vi "PH_SSAC.correct Frames.vi"(0 "i ref in":refnum<vi>, 5 "error in":errorcluster) -> (14 "i ref out":refnum<vi>, 19 "error out":errorcluster)   [LabVIEW 2014, in "PH_SSAC.lvlib"]
doc: "This VI checks the image size and corrects - if necessary - the size of the frames used for the main and the background signal."
uses:
  PH_SSAC.lvlib
  PH_SSAC.Signal Selector.ctl
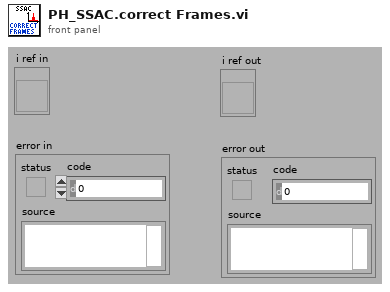
[diagram p1: front panel]
types:
  T1 = typedef "PH_SSAC.lvlib/PH_SSAC.Signal Selector.ctl" = enum16{"Main", "Background"}
  T2 = typedef "PH_SSAC.lvlib/PH_SSAC.i attribute.ctl" = cluster{"GUI Refs":cluster{"Delete":refnum<vi>, "Global On":refnum<vi>, "Cam Source":refnum<vi>, "Frame Main Signal":refnum<vi>, "Frame Background":refnum<vi>, "dt (Gauss smooth)":refnum<vi>, "Calibration Factor":refnum<vi>, "Background acquire":refnum<vi>, "Threshold":refnum<vi>, "Time evolution of mean pulse duration":refnum<vi>, "Mean Pulse Duration":refnum<vi>, "Main signal":refnum<vi>, "Current Pulse Duration":refnum<vi>, "Processed":refnum<vi>, "Saturation":refnum<vi>, "# for Average":refnum<vi>, "Position":refnum<vi>, "BG Status":refnum<vi>, "Save BG data":refnum<vi>, "Read BG Data":refnum<vi>, "Background Calibration Data":refnum<vi>}, "Images":cluster{"OP Image":T3, "GUI Image":T3, "PSDB Image":T3}, "Global On?":bool, "Frame Main":cluster{"x":u32, "dx":u32, "y":u32, "dy":u32}, "Frame Background":cluster{"x":u32, "dx":u32, "y":u32, "dy":u32}, "dt [fs]":dbl, "Calibration Factor [fs/pixel]":dbl, "Threshold":dbl, "Time evolution of mean pulse duration [fs]":dbl[], "Main Signal":cluster{"Time for Main":dbl[], "Signal":dbl[]}, "Processed":bool, "Current Pulse Duration [fs]":dbl, "# for Average":i32, "Position":i32, "Pulse Durations [fs]":dbl[], "BG":cluster{"Acquire?":bool, "Background Calibration Data":T4, "Save Data":bool}}
  T3 = typedef "IMAQ Image.ctl" = refnum<image>
  T4 = typedef "PH_SSAC.lvlib/PH_SSAC.Background Data.ctl" = cluster{"Date":string, "Time":string, "Frame Main":cluster{"x":u32, "dx":u32, "y":u32, "dy":u32}, "dt [fs]":dbl, "Calibration Factor [fs/pixel]":dbl, "Signal":dbl[], "Frame Background":cluster{"x":u32, "dx":u32, "y":u32, "dy":u32}}
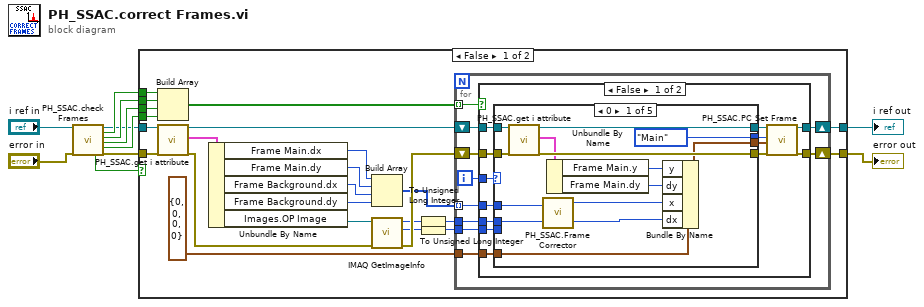
[diagram p0: block diagram]
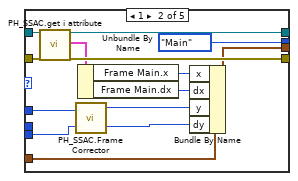
[diagram p2: hidden frame]
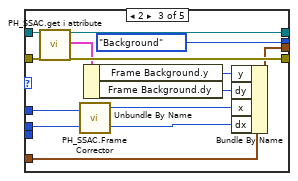
[diagram p3: hidden frame]
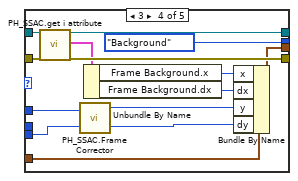
[diagram p4: hidden frame]
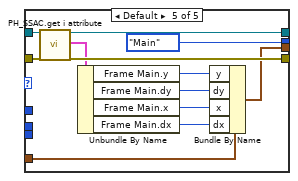
[diagram p5: hidden frame]
diagram:
  n1 = call "PH_SSAC.check Frames.vi"("i ref in"="i ref in", "error in"="error in") -> ("All ok?"=w1:bool, "i ref out"=w2:refnum<vi>, "x Dimension Main ok?"=w9:bool, "y Dimension Main ok?"=w8:bool, "x Dimension Background ok?"=w7:bool, "y Dimension Background ok?"=w6:bool, "error out"=w3:errorcluster)  [unwired: 11 in]
  n2 = case shown="False" w1 {
    tunnel: [w32 w130] -> w11
    tunnel: [w30 w129] -> w10
    tunnel: w9 -> [w20 _]
    tunnel: w8 -> [w19 _]
    tunnel: w7 -> [w18 _]
    tunnel: w6 -> [w17 _]
    tunnel: w3 -> [w16 w129]
    tunnel: w2 -> [w15 w130]
    frame False {
      n3 = Build Array(w20, w19, w18, w17) -> (w33:bool[])
      n4 = call "PH_SSAC.get i attribute.vi"("i ref in"=w15, "error in (no error)"=w16) -> ("i ref out"=w14:refnum<vi>, "i attribute"=w35:T2, "error out"=w13:errorcluster)  [unwired: 15 in]
      n5 = Unbundle By Name(w35) -> ("Frame Main.dx"=w29:u32, "Frame Main.dy"=w23:u32, "Frame Background.dx"=w22:u32, "Frame Background.dy"=w21:u32, "Images.OP Image"=w34:T3)
      n6 = Build Array(w29, w23, w22, w21) -> (w24:u32[])
      n7 = call "IMAQ GetImageInfo"("error in (no error)"=w13, "Image"=w34) -> ("error out"=w31:errorcluster, "Y Resolution"=w27:i32, "X Resolution"=w28:i32)  [unwired: 2 in, 5 out]
      n8 = To Unsigned Long Integer(number=w28) -> (unsigned 32bit integer=w26:u32)
      n9 = To Unsigned Long Integer(number=w27) -> (unsigned 32bit integer=w25:u32)
      n10 = for {
        tunnel: w33 -> [w41] mode=indexing
        shift-right: [w44] -> w32
        shift-left: w14 -> [w45]
        shift-right: [w42] -> w30
        shift-left: w31 -> [w43]
        tunnel: w26 -> [w39]
        tunnel: w24 -> [w38] mode=indexing
        tunnel: w25 -> [w37]
        tunnel: cluster{"x":u32, "dx":u32, "y":u32, "dy":u32} {"x"=0, "dx"=0, "y"=0, "dy"=0} ("Frame") -> [w36]
        i -> [w40]
        n11 = case shown="False" w41 {
          tunnel: w45 -> [w53 w128]
          tunnel: [w58 w128] -> w44
          tunnel: w43 -> [w55 w127]
          tunnel: [w57 w127] -> w42
          tunnel: w40 -> [w51 _]
          tunnel: w39 -> [w49 _]
          tunnel: w38 -> [w48 _]
          tunnel: w37 -> [w47 _]
          tunnel: w36 -> [w46 _]
          frame False {
            n12 = case shown="0" w51 {
              tunnel: [PH_SSAC.Signal_Selector."Main" ("Signal") PH_SSAC.Signal_Selector."Main" ("Signal") PH_SSAC.Signal_Selector."Background" ("Signal") PH_SSAC.Signal_Selector."Background" ("Signal") PH_SSAC.Signal_Selector."Main" ("Signal")] -> w56
              tunnel: w55 -> [w71 w85 w99 w113 w125]
              tunnel: [w70 w84 w98 w112 w124] -> w54
              tunnel: w53 -> [w69 w83 w97 w111 w123]
              tunnel: [w68 w82 w96 w110 w122] -> w52
              tunnel: [w67 w81 w95 w109 w121] -> w50
              tunnel: w49 -> [w62 _ w91 _ _]
              tunnel: w48 -> [w61 w77 w90 w105 _]
              tunnel: w47 -> [_ w76 _ w104 _]
              tunnel: w46 -> [w59 w73 w87 w101 w115]
              frame 0 {
                n13 = call "PH_SSAC.get i attribute.vi"("i ref in"=w69, "error in (no error)"=w71) -> ("i ref out"=w68:refnum<vi>, "i attribute"=w66:T2, "error out"=w70:errorcluster)  [unwired: 15 in]
                n14 = call "PH_SSAC.Frame Corrector.vi"("Image Dimension"=w62, "Frame Dimension"=w61) -> ("Corrected Frame Dimension"=w60:u32, "Corrected Frame Start Point"=w63:u32)
                n15 = Unbundle By Name(w66) -> ("Frame Main.y"=w65:u32, "Frame Main.dy"=w64:u32)
                n16 = Bundle By Name(cluster=w59, "y"=w65, "dy"=w64, "x"=w63, "dx"=w60) -> (w67:cluster{"x":u32, "dx":u32, "y":u32, "dy":u32})
              }
              frame 1 {
                n17 = call "PH_SSAC.get i attribute.vi"("i ref in"=w83, "error in (no error)"=w85) -> ("i ref out"=w82:refnum<vi>, "i attribute"=w80:T2, "error out"=w84:errorcluster)  [unwired: 15 in]
                n18 = call "PH_SSAC.Frame Corrector.vi"("Image Dimension"=w76, "Frame Dimension"=w77) -> ("Corrected Frame Dimension"=w74:u32, "Corrected Frame Start Point"=w75:u32)
                n19 = Unbundle By Name(w80) -> ("Frame Main.x"=w79:u32, "Frame Main.dx"=w78:u32)
                n20 = Bundle By Name(cluster=w73, "x"=w79, "dx"=w78, "y"=w75, "dy"=w74) -> (w81:cluster{"x":u32, "dx":u32, "y":u32, "dy":u32})
              }
              frame 2 {
                n21 = call "PH_SSAC.get i attribute.vi"("i ref in"=w97, "error in (no error)"=w99) -> ("i ref out"=w96:refnum<vi>, "i attribute"=w94:T2, "error out"=w98:errorcluster)  [unwired: 15 in]
                n22 = call "PH_SSAC.Frame Corrector.vi"("Image Dimension"=w91, "Frame Dimension"=w90) -> ("Corrected Frame Dimension"=w88:u32, "Corrected Frame Start Point"=w89:u32)
                n23 = Unbundle By Name(w94) -> ("Frame Background.y"=w93:u32, "Frame Background.dy"=w92:u32)
                n24 = Bundle By Name(cluster=w87, "y"=w93, "dy"=w92, "x"=w89, "dx"=w88) -> (w95:cluster{"x":u32, "dx":u32, "y":u32, "dy":u32})
              }
              frame 3 {
                n25 = call "PH_SSAC.get i attribute.vi"("i ref in"=w111, "error in (no error)"=w113) -> ("i ref out"=w110:refnum<vi>, "i attribute"=w108:T2, "error out"=w112:errorcluster)  [unwired: 15 in]
                n26 = call "PH_SSAC.Frame Corrector.vi"("Image Dimension"=w104, "Frame Dimension"=w105) -> ("Corrected Frame Dimension"=w102:u32, "Corrected Frame Start Point"=w103:u32)
                n27 = Unbundle By Name(w108) -> ("Frame Background.x"=w107:u32, "Frame Background.dx"=w106:u32)
                n28 = Bundle By Name(cluster=w101, "x"=w107, "dx"=w106, "y"=w103, "dy"=w102) -> (w109:cluster{"x":u32, "dx":u32, "y":u32, "dy":u32})
              }
              frame Default {
                n29 = call "PH_SSAC.get i attribute.vi"("i ref in"=w123, "error in (no error)"=w125) -> ("i ref out"=w122:refnum<vi>, "i attribute"=w120:T2, "error out"=w124:errorcluster)  [unwired: 15 in]
                n30 = Unbundle By Name(w120) -> ("Frame Main.y"=w119:u32, "Frame Main.dy"=w118:u32, "Frame Main.x"=w117:u32, "Frame Main.dx"=w116:u32)
                n31 = Bundle By Name(cluster=w115, "y"=w119, "dy"=w118, "x"=w117, "dx"=w116) -> (w121:cluster{"x":u32, "dx":u32, "y":u32, "dy":u32})
              }
            }
            n32 = call "PH_SSAC.PC Set Frame.vi"("i ref in"=w52, "Signal"=w56, "Frame"=w50, "error IO"=w54) -> ("i ref out"=w58:refnum<vi>, "error out"=w57:errorcluster)  [unwired: 14 in]
          }
          frame True {
          }
        }
      }
    }
    frame True {
    }
  }
  "i ref out" <- w11
  "error out" <- w10
